vi "trial code 2.vi"() -> ()   [LabVIEW 2025]
uses:
  <vilib>/Instr/_visa.llb/VISA Configure Serial Port (Instr).vi
  <vilib>/addons/control/pid/NI_PID_pid.lvlib
  <vilib>/addons/control/pid/pid.llb/PID (DBL).vi
panel:
  out "Read Heave and Surge":string
  out "Instrument Status":bool
  out "LastCom":string
  in  "WriteCC1 2":string[](array[string])=[""]
  out "Error Heave":errorcluster
  out "Heave COM Status 3":bool
  in  "Enum":enum16{"init", "MAIN", "Panel Close"}(ring)
  in  "Write S":bool
  in  "String 36":string
  in  "Com Port 3":refnum<visa-resource-name>="COM7" caption="COM Port Heave :"
  out "Bytes at Heave Port":dbl
  out "Port 5":bool=TRUE caption="Port 2"
  in  "Heave PPR":dbl=6400.0
  in  "Sway PPR":dbl=6400.0
  in  "Surge PPR":dbl=6400.0
  in  "Heave Pitch":dbl=4.0
  in  "Sway Pitch":dbl=2.0
  in  "Surge Pitch":dbl=3.0
  out "Sway Pulses/mm":dbl=320.0
  out "Surge Pulses/mm":dbl=1600.0
  out "Heave Pulses/mm":dbl=1600.0
  in  "Test Method":u16(ring) items=["Erosion Tester", "Double Disc"]
  in  "input variable":dbl=1.0
  out "output Vpp":dbl
  out "output variable":dbl
  in  "Stop 3":bool
  in  "PID ON":bool
  out "Stroke":dbl
  in  "Stop 2":bool
  in  "PID SEND":bool
  in  "Set Strk":dbl=1.0 caption="STROKE LENGTH" min=1.0 max=1.0 step=1.0 format="%.3f"
  in  "PID Rst":bool=TRUE
  out "Stroke PID OUT":dbl(slide)=-13.483146067415703 scale=-600.0..600.0
  out "stop cmd":bool
  out "st gain":string="0000"
  out "PID Out":u8(slide) scale=0.0..4095.0
  in  "Stroke PID Gains 2":T1={"Proportional Gain (Kc)"=200.0, "Integral Time (Ti, min)"=0.02, "Derivative Time (Td, min)"=0.0}
  out "start en":bool=TRUE
  in  "STROKE GAIN :":dbl=700.0 caption="Stroke Gain :"
  out "Residual Uno 2":string
  out "Port 1 Error 2":errorcluster={"status"=TRUE, "code"=-1073807343, "source"="Property Node (arg 1) in VISA Configure Serial Port (Instr).vi->Winducom 2010--std ed hfrr-wo1768-V18.vi"}
  out "Sps 4":dbl
  out "Port 1a 2":bool caption="Port 1 a"
  out "Port 2":u32(graph)
  out "Uno Stroke":string
  out "LVDT MIN":dbl
  out "LVDT MAX":dbl
  out "LVDT Peak":dbl
  out "pizo raw":dbl
  out "Friction":dbl
  out "cof":dbl
  out "Error Uno 2":errorcluster={"status"=TRUE, "code"=-1073807343, "source"="Property Node (arg 1) in VISA Configure Serial Port (Instr).vi->Winducom 2010--std ed hfrr-wo1768-V18.vi"}
  out "Port 4":bool=TRUE caption="Port 1"
  in  "Re-initialize Port1 2":bool
  in  "Com Port 2":refnum<visa-resource-name>="COM9" caption="C2 :"
  out "Residual Uno":string
  out "Port 1 Error":errorcluster={"status"=TRUE, "code"=-1073807343, "source"="Property Node (arg 1) in VISA Configure Serial Port (Instr).vi->Winducom 2010--std ed hfrr-wo1768-V18.vi"}
  out "due":string
  out "Sps 3":dbl
  out "Port 1a":bool caption="Port 1 a"
  out "Port 1":u32(graph)
  out "Error Uno":errorcluster={"status"=TRUE, "code"=-1073807343, "source"="Property Node (arg 1) in VISA Configure Serial Port (Instr).vi->Winducom 2010--std ed hfrr-wo1768-V18.vi"}
  out "Port 3":bool=TRUE caption="Port 1"
  in  "Re-initialize Port1":bool
  in  "Stop":bool
  in  "command":string
  out "FF buffer":dbl[](graph)
  in  "Com Port 1":refnum<visa-resource-name>="COM7" caption="C1 :"
  out "Test \nStatus":bool caption="Test Status"
types:
  T1 = cluster{"Proportional Gain (Kc)":dbl, "Integral Time (Ti, min)":dbl, "Derivative Time (Td, min)":dbl}
  T2 = cluster{"Read Heave and Surge":string, "Bytes at Heave Port":dbl, "Heave and Surge COM Port:":refnum<visa-resource-name>, "Com Port 2":refnum<visa-resource-name>, "Residual Due":string, "Heave COM Status 2":bool, "Heave COM Status":bool, "Port 2":bool, "Sway PPR":dbl, "Surge PPR":dbl, "Heave PPR":dbl, "Sway Pitch":dbl, "Surge Pitch":dbl, "Heave Pitch":dbl, "Sway Pulses/mm":dbl, "Surge Pulses/mm":dbl, "Heave Pulses/mm":dbl, "inner loop":dbl, "Read Heave and Surge 2":string, "String 36":string, "Write S":bool, "WriteCC1":string[], "Heave COM Loop":i32, "LastCom":string, "EXIT":bool, "Error Heave":errorcluster}
  T3 = enum16{"INIT", "READ", "MANUAL WRITE", "WRITE", "CLOSE", "ERROR INIT"}
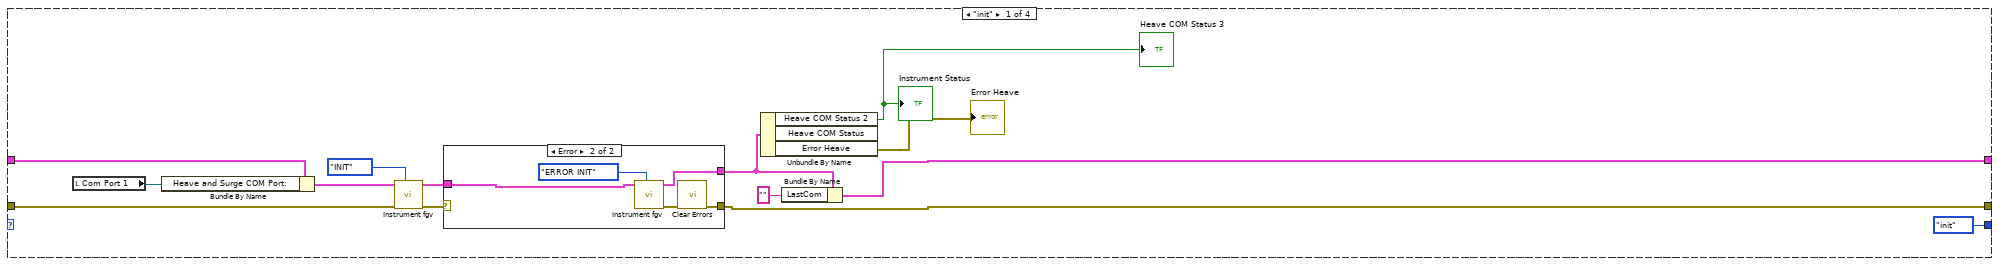
[diagram p2: hidden frame]
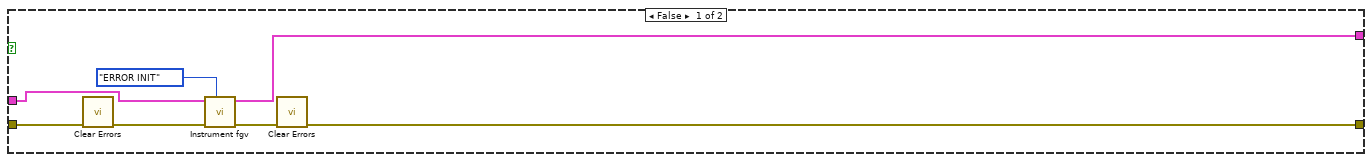
[diagram p4: hidden frame]
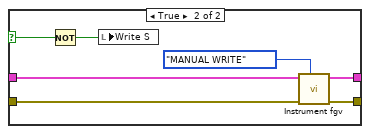
[diagram p7: hidden frame]
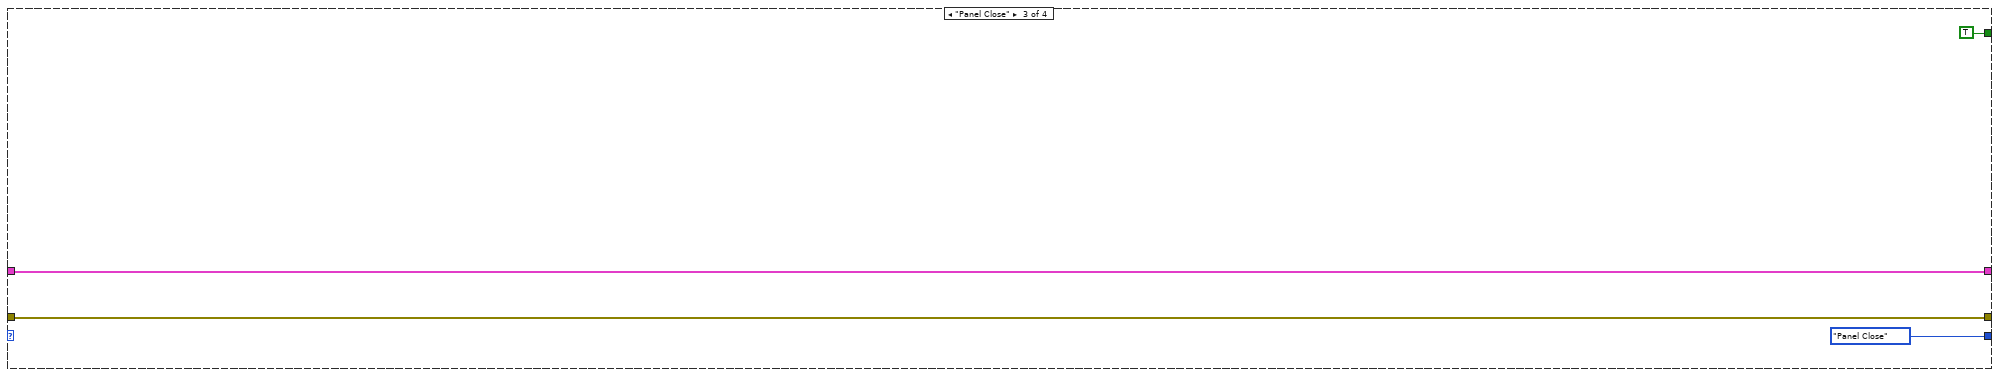
[diagram p8: hidden frame]
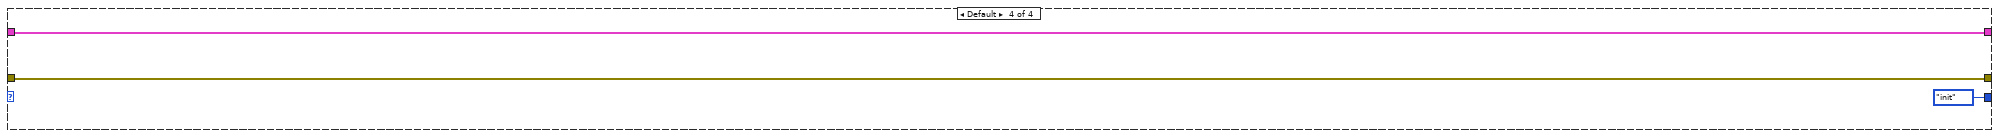
[diagram p9: hidden frame]
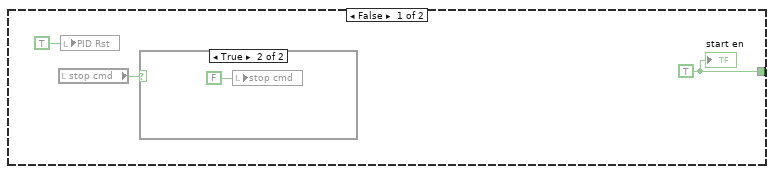
[diagram p13: hidden frame]
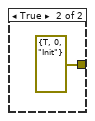
[diagram p19: hidden frame]
diagram:
  # "lvdt min,lvdt max,lvdt peak,pizo raw data , friction netwon ,cof"
  n1 = while {
    shift-right: [w12] -> _
    shift-left: _ -> [w8]
    shift-right: [w10] -> _
    shift-left: T2 {"Read Heave and Surge"="", "Bytes at Heave Port"=0.0, "Heave and Surge COM Port:"="COM9", "Com Port 2"="COM7", "Residual Due"="", "Heave COM Status 2"=TRUE, "Heave COM Status"=TRUE, "Port 2"=TRUE, "Sway PPR"=6400.0, "Surge PPR"=6400.0, "Heave PPR"=6400.0, "Sway Pitch"=2.0, "Surge Pitch"=3.0, "Heave Pitch"=4.0, "Sway Pulses/mm"=320.0, "Surge Pulses/mm"=1600.0, "Heave Pulses/mm"=1600.0, "inner loop"=0.0, "Read Heave and Surge 2"="", "String 36"="", "Write S"=FALSE, "WriteCC1"=[""], "Heave COM Loop"=0, "LastCom"="", "EXIT"=FALSE, "Error Heave"={"status"=TRUE, "code"=-1073807343, "source"=""}} -> [w9]
    shift-right: [w6] -> _
    shift-left: "Enum" -> [w7]
    stop <- w11 stop-if-true
    n2 = case shown="\"MAIN\"" w7 {
      tunnel: w8 -> [w26 w41 w109 w112]
      tunnel: [w21 w56 w109 w112] -> w12
      tunnel: [_ _ TRUE _] -> w11
      tunnel: [w17 w53 w107 w111] -> w10
      tunnel: w9 -> [w23 w40 w107 w111]
      tunnel: [enum16{"init", "MAIN", "Panel Close"}."init" ("Enum") enum16{"init", "MAIN", "Panel Close"}."MAIN" ("Enum") enum16{"init", "MAIN", "Panel Close"}."Panel Close" ("Enum") enum16{"init", "MAIN", "Panel Close"}."init" ("Enum")] -> w6
      frame "init" {
        n3 = local read "Com Port 1"() -> (w15:refnum<visa-resource-name>)
        n4 = Bundle By Name(cluster=w23, "Heave and Surge COM Port:"=w15) -> (w22:T2)
        n5 = call "Instrument fgv.vi"("Enum"=T3."INIT", "error in (no error) 2"=w26, "INPUT"=w22) -> ("error"=w24:errorcluster, "output"=w20:T2)  [unwired: 6 in, 1 out]
        n6 = case shown="Error" w24 {
          selector: w24 -> [w28 _]
          tunnel: [w28 w32] -> w21
          tunnel: w20 -> [w27 w30]
          tunnel: [w27 w29] -> w18
          frame No Error {
          }
          frame Error {
            n7 = call "Instrument fgv.vi"("Enum"=T3."ERROR INIT", "INPUT"=w30) -> ("error"=w33:errorcluster, "output"=w29:T2)  [unwired: 7 in, 1 out]
            n8 = call <vilib>:"Clear Errors.vi"("error in (no error)"=w33) -> ("error out"=w32:errorcluster)  [unwired: 5 in, 1 out]
          }
        }
        n9 = Unbundle By Name(w18) -> ("Heave COM Status 2"=→"Heave COM Status 3" →"Instrument Status":bool, "Error Heave"=→"Error Heave":errorcluster)  [unwired: 1 out]
        n10 = Bundle By Name(cluster=w18, "LastCom"="") -> (w17:T2)
      }
      frame "MAIN" {
        n11 = Unbundle By Name(w40) -> ("Com Port 2"=w58:refnum<visa-resource-name>)
        n12 = local read "Com Port 1"() -> (w37:refnum<visa-resource-name>)
        n13 = local write "Com Port 3"(w58) -> ()
        n14 = Bundle By Name(cluster=w40, "Heave and Surge COM Port:"=w37) -> (w39:T2)
        n15 = Equal?(x=w58, y=w37) -> (x = y?=w57:bool)
        n16 = Divide(x="Heave PPR", y="Heave Pitch") -> (x/y=→"Heave Pulses/mm":dbl)
        n17 = case shown="True" w57 {
          tunnel: [w62 w79] -> w56
          tunnel: w41 -> [w63 w85]
          tunnel: w39 -> [w61 w83]
          tunnel: [w60 w78] -> w53
          frame False {
            n18 = call <vilib>:"Clear Errors.vi"("error in (no error)"=w63) -> ("error out"=w59:errorcluster)  [unwired: 5 in, 1 out]
            n19 = call "Instrument fgv.vi"("Enum"=T3."ERROR INIT", "error in (no error) 2"=w59, "INPUT"=w61) -> ("error"=w65:errorcluster, "output"=w60:T2)  [unwired: 6 in, 1 out]
            n20 = call <vilib>:"Clear Errors.vi"("error in (no error)"=w65) -> ("error out"=w62:errorcluster)  [unwired: 5 in, 1 out]
          }
          frame True {
            n21 = call "Instrument fgv.vi"("Enum"=T3."READ", "error in (no error) 2"=w85, "INPUT"=w83) -> ("error"=w84:errorcluster, "output"=w76:T2)  [unwired: 6 in, 1 out]
            n22 = Bundle By Name(cluster=w76, "String 36"="String 36") -> (w75:T2)
            n23 = case shown="False" "Write S" {
              selector: "Write S" -> [_ w105]
              tunnel: w84 -> [w98 w104]
              tunnel: [w98 w103] -> w73
              tunnel: w75 -> [w97 w100]
              tunnel: [w97 w99] -> w72
              frame False {
              }
              frame True {
                n24 = Not(x=w105) -> (.not. x?=w101:bool)
                n25 = local write "Write S"(w101) -> ()
                n26 = call "Instrument fgv.vi"("Enum"=T3."MANUAL WRITE", "error in (no error) 2"=w104, "INPUT"=w100) -> ("error"=w103:errorcluster, "output"=w99:T2)  [unwired: 6 in, 1 out]
              }
            }
            n27 = Array Size(array="WriteCC1 2") -> (size(s)=w70:i32)
            n28 = Greater Than 0?(x=w70) -> (x > 0?=w69:bool)
            n29 = call "Instrument fgv.vi"("Enum"=T3."WRITE", "error in (no error) 2"=w73, "WriteCC1"="WriteCC1 2", "INPUT"=w72) -> ("error"=w81:errorcluster, "WriteCC1 2"=w71:string[], "output"=w80:T2)  [unwired: 5 in]
            n30 = case shown="True" w69 {
              tunnel: w71 -> [_ w87]
              frame False {
              }
              frame True {
                n31 = local write "WriteCC1 2"(w87) -> ()
              }
            }
            n32 = case shown="Error" w81 {
              selector: w81 -> [w88 w91]
              tunnel: w80 -> [w89 w96]
              tunnel: [w89 w95] -> w78
              tunnel: [w88 w93] -> w79
              frame No Error {
              }
              frame Error {
                n33 = call <vilib>:"Clear Errors.vi"("error in (no error)"=w91) -> ("error out"=w90:errorcluster)  [unwired: 5 in, 1 out]
                n34 = call "Instrument fgv.vi"("Enum"=T3."ERROR INIT", "error in (no error) 2"=w90, "INPUT"=w96) -> ("error"=w94:errorcluster, "output"=w95:T2)  [unwired: 6 in, 1 out]
                n35 = call <vilib>:"Clear Errors.vi"("error in (no error)"=w94) -> ("error out"=w93:errorcluster)  [unwired: 5 in, 1 out]
              }
            }
            n36 = Unbundle By Name(w78) -> ("LastCom"=→"LastCom":string, "Read Heave and Surge"=→"Read Heave and Surge":string)
          }
        }
        n37 = Divide(x="Sway PPR", y="Sway Pitch") -> (x/y=→"Sway Pulses/mm":dbl)
        n38 = Divide(x="Surge PPR", y="Surge Pitch") -> (x/y=→"Surge Pulses/mm":dbl)
        n39 = Unbundle By Name(w53) -> ("Heave COM Status 2"=w55:bool, "Heave COM Status"=w54:bool, "Error Heave"=w35:errorcluster, "Bytes at Heave Port"=→"Bytes at Heave Port":dbl)
        n40 = Unbundle By Name(w35) -> ("status"=→"Port 5":bool)
        n41 = Not(x=w54) -> (.not. x?=w34:bool)
        n42 = Not(x=w55) -> (.not. x?=w36:bool)
        n43 = local write "Instrument Status"(w34) -> ()
        n44 = local write "Heave COM Status 3"(w36) -> ()
        n45 = local write "Error Heave"(w35) -> ()
      }
      frame "Panel Close" {
      }
      frame Default {
      }
    }
  }
  n46 = disable-structure shown="Disabled" {
    frame Disabled {
      n47 = case shown="True" {
        selector: _ -> [_ _]
        tunnel: [w113 _] -> _
        frame False {
          w113 = TRUE ("PID Rst")
          n48 = local read "stop cmd"() -> (w114:bool)
          n49 = local write "PID Rst"(TRUE ("PID Rst")) -> ()
          n50 = case shown="True" w114 {
            frame False {
            }
            frame True {
              n51 = local write "stop cmd"(FALSE ("stop cmd")) -> ()
            }
          }
          "start en" <- w113
        }
        frame True {
          w133 = cluster{"output high":dbl, "output low":dbl} {"output high"=600.0, "output low"=-600.0} ("output range")
          n52 = local read "STROKE GAIN :"() -> (w123:dbl)
          n53 = call "Elapsed Time"("Reset"="PID Rst", "Auto Reset"=FALSE) -> ("Time has Elapsed"=w130:bool)  [unwired: 10 in, 7 out]
          n54 = Unbundle(w133) -> ()  [unwired: 2 out]
          n55 = Select(t=T1 {"Proportional Gain (Kc)"=0.0, "Integral Time (Ti, min)"=0.02, "Derivative Time (Td, min)"=0.0} ("Stroke PID Gains"), f="Stroke PID Gains 2") -> (s? t:f=w120:T1)  [unwired: 1 in]
          n56 = Not(x=w130) -> (.not. x?=w129:bool)
          n57 = Multiply(x="Set Strk", y=w123) -> (x*y=w118:dbl)
          n58 = call-poly <vilib>:"PID.vi"("reinitialize? (F)"=w129, "output range"=w133, "PID gains"=w120, "process variable"="Set Strk", "setpoint"="Set Strk") -> ("output"=w128:dbl)  [unwired: 5 in, 1 out]
          "Stroke PID OUT" <- w128
          n59 = Multiply(x=w118, y=1.0) -> ()  [unwired: 1 out]
          n60 = Select(t=w128, s=w130, f=0.0) -> (s? t:f=w131:dbl)
          n61 = To Word Integer(number=w131) -> (16bit integer=w125:i16)
          n62 = flat-sequence {
            tunnel: w131 -> [_]
            frame #0 {
              n63 = local write "PID Rst"(FALSE ("PID Rst")) -> ()
            }
          }
          n64 = In Range and Coerce(upper limit=0.52 ("f"), x=w125, lower limit=0.49 ("f")) -> (coerced(x)=w122:dbl)  [unwired: 1 out]
          "PID Out" <- w122
          n65 = Number To Decimal String(number=w122) -> (decimal integer string=→"st gain":string)  [unwired: 1 in]
          "stop cmd" <- TRUE ("Auto Reset")
        }
      }
    }
    frame Enabled {
    }
  }
  n66 = while {
    shift-right: [w142] -> _
    shift-left: _ -> [w152]
    shift-right: [w143] -> _
    shift-left: _ -> [w154]
    tunnel: [w156] -> _
    i -> [w156]
    stop <- "Stop" stop-if-true
    n67 = local read "Com Port 1"() -> (w153:refnum<visa-resource-name>)
    n68 = Unbundle(w154) -> ("status"=→"Port 3":bool)  [unwired: 2 out]
    n69 = Not Equal?(x=w153, y=w152) -> (x != y?=w151:bool)
    n70 = Or(x=w151, y="Re-initialize Port1") -> (x .or. y?=w149:bool)
    n71 = case shown="False" w149 {
      tunnel: [w171 errorcluster {"status"=TRUE, "code"=0, "source"="Init"} ("error out")] -> w150
      tunnel: w154 -> [w171 _]
      frame False {
      }
      frame True {
      }
    }
    n72 = call <vilib>:"High Resolution Polling Wait.vi"("seconds to wait"=1.0) -> ()  [unwired: 10 in, 1 out]
    n73 = case shown="No Error" w150 {
      selector: w150 -> [w179 w209]
      tunnel: [w182 w213] -> w144
      tunnel: [w181 w206] -> w145
      tunnel: w152 -> [w180 w211]
      frame No Error {
        n74 = property class="Instr"(reference=w180, error in=w179) -> (reference out=w177:refnum<visa-resource-name>, error out=w178:errorcluster, "Serial Settings:Number of Bytes at Serial Port"=w173:u32)
        "Sps 3" <- w173
        "Port 1" <- w173
        n75 = Greater?(x=w173, y=u32 5) -> (0:w175:bool)
        n76 = Not(x=w175) -> (.not. x?=→"Port 1a":bool)
        n77 = case shown="True" w175 {
          tunnel: w177 -> [w184 w188]
          tunnel: w178 -> [w183 w186]
          tunnel: [w183 w185] -> w181
          tunnel: [w184 w189] -> w182
          frame False {
          }
          frame True {
            (unwired) TRUE ("PAUSE")
            n78 = local read "Residual Uno"() -> (w187:string)
            n79 = while {
              tunnel: [w201] -> w185
              tunnel: [w200] -> w189
              tunnel: w186 -> [w199]
              tunnel: w188 -> [w198]
              tunnel: [w196] -> _
              shift-right: [w193] -> _
              shift-left: w187 -> [w194]
              i -> [w196]
              stop <- TRUE stop-if-true
              n80 = property class="Instr"(reference=w198, error in=w199) -> (reference out=w203:refnum<visa-resource-name>, error out=w202:errorcluster, "Serial Settings:Number of Bytes at Serial Port"=w195:u32)
              n81 = Greater?(x=w195, y=u32 30) -> ()  [unwired: 1 out]
              n82 = VISA Read(VISA resource name=w203, byte count=u32 1000, error in (no error)=w202) -> (VISA resource name out=w200:refnum<visa-resource-name>, read buffer=w190:string, error out=w201:errorcluster)  [unwired: 1 out]
              "due" <- w190
              n83 = Concatenate Strings(w194, w190) -> (w193:string)
            }
          }
        }
      }
      frame Error {
        w219 = u16 0 items=["None", "XON/XOFF", "RTS/CTS", "XON/XOFF & RTS/CTS", "DTR/DSR", "XON/XOFF & DTR/DSR"] ("flow control (0:none)  2")
        w217 = u16 10 items=["1.0"=10, "1.5"=15, "2.0"=20] ("stop bits 2")
        w215 = u16 0 items=["None", "Odd", "Even", "Mark", "Space"] ("parity 2")
        w216 = u32 10000  # timeout (10sec)
        n84 = VISA Close(VISA resource name=w211, error in (no error)=w209) -> (error out=w212:errorcluster)
        n85 = local write "Sps 3"(0.0 ("Sps 4")) -> ()
        n86 = local write "Port 1a"(FALSE ("Port 1a")) -> ()
        n87 = call <vilib>:"Clear Errors.vi"("error in (no error)"=w212) -> ("error out"=w210:errorcluster)  [unwired: 5 in, 1 out]
        n88 = local read "Com Port 1"() -> (w205:refnum<visa-resource-name>)
        n89 = call-poly "VISA Configure Serial Port"("VISA resource name"=w205, "timeout (10sec)"=w216, "baud rate (9600)"=u32 250000 ("baud rate  2"), "data bits (8)"=u16 8 ("data bits  2"), "parity (0:none)"=w215, "error in (no error)"=w210, "stop bits (10: 1 bit)"=w217, "flow control (0:none)"=w219) -> ("VISA resource name out"=w220:refnum<visa-resource-name>, "error out"=w221:errorcluster)  [unwired: 6 in]
        n90 = flat-sequence {
          tunnel: w220 -> [w223]
          tunnel: w221 -> [w222]
          tunnel: [w223] -> w213
          tunnel: [w222] -> w206
          frame #0 {
            n91 = Wait (ms)(milliseconds to wait=u32 50) -> ()  [unwired: 1 out]
          }
        }
        "Residual Uno" <- ""
        "Port 1 Error" <- w206
      }
    }
    n92 = Not Equal?(x="command", y="") -> (x != y?=w140:bool)
    n93 = case shown="True" w140 {
      tunnel: w144 -> [w158 w163]
      tunnel: [w158 w167] -> w142
      tunnel: w145 -> [w157 w162]
      tunnel: [w157 w165] -> w143
      tunnel: "command" -> [_ w161]
      tunnel: [_ w164] -> _
      frame False {
        # "DATA  WRITE LOOP"
      }
      frame True {
        n94 = Concatenate Strings(w161, "\r\n") -> (w160:string)
        n95 = VISA Write(VISA resource name=w163, write buffer=w160, error in (no error)=w162) -> (VISA resource name out=w167:refnum<visa-resource-name>, return count=w164:u32, error out=w166:errorcluster)
        n96 = flat-sequence {
          tunnel: w166 -> [w169]
          tunnel: [w169] -> w165
          frame #0 {
            n97 = local write "command"("" ("command")) -> ()
            n98 = Wait (ms)(milliseconds to wait=u32 5) -> ()  [unwired: 1 out]
          }
        }
      }
    }
    "Error Uno" <- w154
  }
  n99 = while {
    shift-right: [w236] -> _
    shift-left: _ -> [w231]
    shift-right: [w235] -> _
    shift-left: _ -> [w232]
    tunnel: [w234] -> _
    i -> [w234]
    stop <- w225 stop-if-true
    n100 = Not Equal?(x="Com Port 2", y=w231) -> (x != y?=w230:bool)
    n101 = Unbundle(w232) -> ("status"=→"Port 4":bool)  [unwired: 2 out]
    n102 = Or(x=w230, y="Re-initialize Port1 2") -> (x .or. y?=w228:bool)
    n103 = case shown="False" w228 {
      tunnel: [w237 errorcluster {"status"=TRUE, "code"=0, "source"="Init"} ("error out")] -> w229
      tunnel: w232 -> [w237 _]
      frame False {
      }
      frame True {
      }
    }
    n104 = case shown="No Error" w229 {
      selector: w229 -> [w245 w276]
      tunnel: [w248 w280] -> w236
      tunnel: [w247 w273] -> w235
      tunnel: w231 -> [w246 w278]
      frame No Error {
        n105 = property class="Instr"(reference=w246, error in=w245) -> (reference out=w243:refnum<visa-resource-name>, error out=w244:errorcluster, "Serial Settings:Number of Bytes at Serial Port"=w239:u32)
        "Sps 4" <- w239
        "Port 2" <- w239
        n106 = Greater?(x=w239, y=u32 5) -> (0:w241:bool)
        n107 = Not(x=w241) -> (.not. x?=→"Port 1a 2":bool)
        n108 = while {
          tunnel: [w268] -> w247
          tunnel: [w267] -> w248
          tunnel: w244 -> [w266]
          tunnel: w243 -> [w265]
          tunnel: [w263] -> _
          i -> [w263]
          stop <- TRUE stop-if-true
          n109 = property class="Instr"(reference=w265, error in=w266) -> (reference out=w270:refnum<visa-resource-name>, error out=w269:errorcluster, "Serial Settings:Number of Bytes at Serial Port"=w262:u32)
          n110 = Greater?(x=w262, y=u32 30) -> ()  [unwired: 1 out]
          n111 = VISA Read(VISA resource name=w270, byte count=u32 1000, error in (no error)=w269) -> (VISA resource name out=w267:refnum<visa-resource-name>, read buffer=w259:string, error out=w268:errorcluster)  [unwired: 1 out]
          "Uno Stroke" <- w259
          n112 = Spreadsheet String To Array(delimiter (Tab)=";", format string="", spreadsheet string=w259, array type (2D Dbl)=dbl[] []) -> (array=w256:dbl[])
          n113 = Index Array(array=w256) -> (element #1=→"LVDT MIN":dbl, element #2=→"LVDT MAX":dbl, element #3=→"LVDT Peak":dbl, element #4=→"pizo raw":dbl, element #5=→"Friction":dbl, element #6=→"cof":dbl)  [unwired: 6 in]
        }
      }
      frame Error {
        w286 = u16 0 items=["None", "XON/XOFF", "RTS/CTS", "XON/XOFF & RTS/CTS", "DTR/DSR", "XON/XOFF & DTR/DSR"] ("flow control (0:none)  2")
        w284 = u16 10 items=["1.0"=10, "1.5"=15, "2.0"=20] ("stop bits 2")
        w282 = u16 0 items=["None", "Odd", "Even", "Mark", "Space"] ("parity 2")
        w283 = u32 10000  # timeout (10sec)
        n114 = VISA Close(VISA resource name=w278, error in (no error)=w276) -> (error out=w279:errorcluster)
        n115 = local write "Sps 4"(0.0 ("Sps 4")) -> ()
        n116 = local write "Port 1a 2"(FALSE ("Port 1a")) -> ()
        n117 = call <vilib>:"Clear Errors.vi"("error in (no error)"=w279) -> ("error out"=w277:errorcluster)  [unwired: 5 in, 1 out]
        n118 = local read "Com Port 2"() -> (w271:refnum<visa-resource-name>)
        n119 = call-poly "VISA Configure Serial Port"("VISA resource name"=w271, "timeout (10sec)"=w283, "baud rate (9600)"=u32 250000 ("baud rate  2"), "data bits (8)"=u16 8 ("data bits  2"), "parity (0:none)"=w282, "error in (no error)"=w277, "stop bits (10: 1 bit)"=w284, "flow control (0:none)"=w286) -> ("VISA resource name out"=w287:refnum<visa-resource-name>, "error out"=w288:errorcluster)  [unwired: 6 in]
        n120 = flat-sequence {
          tunnel: w287 -> [w290]
          tunnel: w288 -> [w289]
          tunnel: [w290] -> w280
          tunnel: [w289] -> w273
          frame #0 {
            n121 = Wait (ms)(milliseconds to wait=u32 50) -> ()  [unwired: 1 out]
          }
        }
        "Residual Uno 2" <- ""
        "Port 1 Error 2" <- w273
      }
    }
    n122 = local read "Stop"() -> (w225:bool)
    "Error Uno 2" <- w232
  }
  n123 = disable-structure shown="Disabled" {
    frame Disabled {
      n124 = while {
        stop <- _ stop-if-true
        n125 = Interpolate 1D Array(2:dbl[] [0.554, 1.041, 1.05, 1.06, 1.071, 1.083, 1.095, 1.11, 1.255] ("array of numbers or points")) -> ()  [unwired: 1 in, 1 out]
      }
    }
    frame Enabled {
    }
  }
  n126 = while {
    stop <- "Stop 2" stop-if-true
    n127 = case shown="True" "PID SEND" {
      selector: "PID SEND" -> [_ w299]
      frame False {
      }
      frame True {
        n128 = Not(x=w299) -> (.not. x?=w298:bool)
        n129 = local write "command"("1" ("command")) -> ()
        n130 = local write "PID SEND"(w298) -> ()
      }
    }
    n131 = local read "LVDT Peak"() -> (w296:dbl)
    n132 = formula code="if (vpp_val <= 0.554) {\n    stroke = 0.5;\n} \nelse if (vpp_val >= 1.255) {\n    stroke = 1.2;\n} \nelse if (vpp_val < 1.041) {\n    stroke = 0.5 + (vpp_val - 0.554) * (0.97 - 0.5) / (1.041 - 0.554);\n} \nelse if (vpp_val < 1.05) {\n    stroke = 0.97 + (vpp_val - 1.041) * (0.98 - 0.97) / (1.05 - 1.041);\n} \nelse if (vpp_val < 1.06) {\n    stroke = 0.98 + (vpp_val - 1.05) * (0.99 - 0.98) / (1.06 - 1.05);\n} \nelse if (vpp_val < 1.071) {\n    stroke = 0.99 + (vpp_val - 1.06) * (1.0 - 0.99) / (1.071 - 1.06);\n} \nelse if (vpp_val < 1.083) {\n    stroke = 1.0 + (vpp_val - 1.071) * (1.01 - 1.0) / (1.083 - 1.071);\n} \nelse if (vpp_val < 1.095) {\n    stroke = 1.01 + (vpp_val - 1.083) * (1.02 - 1.01) / (1.095 - 1.083);\n} \nelse if (vpp_val < 1.11) {\n    stroke = 1.02 + (vpp_val - 1.095) * (1.04 - 1.02) / (1.11 - 1.095);\n} \nelse {\n    stroke = 1.04 + (vpp_val - 1.11) * (1.2 - 1.04) / (1.255 - 1.11);\n}"("vpp_val"=w296) -> ("stroke"=→"Stroke":dbl)
  }
  n133 = while {
    shift-right: [w305] -> _
    shift-left: 0.0 -> [w307]
    shift-right: [w304] -> _
    shift-left: 0.0 -> [w306]
    shift-right: [w302] -> _
    shift-left: 400.0 ("vc_cmd") -> [w303]
    stop <- "Stop 3" stop-if-true
    n134 = case shown="True" "PID ON" {
      tunnel: w307 -> [w310 w318]
      tunnel: w306 -> [w309 w317]
      tunnel: [w310 w316] -> w305
      tunnel: [w309 w315] -> w304
      tunnel: w303 -> [w308 w313]
      tunnel: [w308 w312] -> w302
      frame False {
      }
      frame True {
        n135 = local read "Stroke"() -> (w320:dbl)
        n136 = Wait (ms)(milliseconds to wait=u32 0) -> ()  [unwired: 1 out]
        n137 = formula code="// 1. Define PID Tuning constants and limits from script\nfloat kp = 2000.0;\nfloat ki = 1300.0;\nfloat kd = 140.0;\nfloat startup_cmd = 400.0;\nfloat max_step_change = 150.0;\nfloat max_amplitude = 1000.0;\nfloat min_amplitude = 0.0;\n\nfloat current_error = 0.0;\nfloat current_integral = 0.0;\nfloat current_derivative = 0.0;\nfloat ideal_command = 0.0;\nfloat raw_adjustment = 0.0;\nfloat adjustment = 0.0;\n\n// 2. Calculate Tracking Error\ncurrent_error = target_stroke - measured_stroke;\nerror_out = current_error; // Output for monitoring\n\n// 3. Calculate Integral and Derivative components\ncurrent_integral = prev_integral_err + (current_error * dt);\ncurrent_derivative = (current_error - prev_error) / dt;\n\n// 4. Compute Ideal PID Target Command\nideal_command = startup_cmd + (kp * current_error) + (ki * current_integral) + (kd * current_derivative);\n\n// 5. Rate Limiting (Enforce MAX_STEP_CHANGE)\nraw_adjustment = ideal_command - prev_vc_cmd;\n\nif (raw_adjustment > max_step_change) {\n    adjustment = max_step_change;\n} else if (raw_adjustment < -max_step_change) {\n    adjustment = -max_step_change;\n} else {\n    adjustment = raw_adjustment;\n}\n\n// Apply the rate-limited adjustment to the previous command\nvc_cmd = prev_vc_cmd + adjustment;\n\n// 6. Output Clamping & Anti-Windup Logic\nif (vc_cmd > max_amplitude) {\n    vc_cmd = max_amplitude;\n    current_integral = current_integral - (current_error * dt); // Undo integral step\n} else if (vc_cmd < min_amplitude) {\n    vc_cmd = min_amplitude;\n    current_integral = current_integral - (current_error * dt); // Undo integral step\n}\n\n// 7. Map local variables to output terminals linked to shift registers\nout_integral_err = current_integral;\nout_error = current_error;"("target_stroke"="input variable", "measured_stroke"=w320, "dt"=0.05 ("input variable"), "prev_integral_err"=w318, "prev_error"=w317, "prev_vc_cmd"=w313) -> ("vc_cmd"=w312:dbl, "out_integral_err"=w316:dbl, "out_error"=w315:dbl, "error_out"=→"output variable":dbl)
        "output Vpp" <- w312
      }
    }
  }
